vi "Open.vi"(8 "error in":errorcluster, 9 "parameters":variant, 10 "file path":path, 11 "cRIO repo in":refnum<class "cRIORepo.lvclass">) -> (0 "error out":errorcluster, 2 "invalid?":bool, 3 "cRIO repo out":refnum<class "cRIORepo.lvclass">)   [LabVIEW 2015, in "cRIORepo.lvclass"]
doc: "Here we are specifying to read the configuration from a gXML file. And version management"
uses:
  cRIORepo.lvclass
  FileCluster.ctl
  ChannelData.ctl
  cRIORepo.lvclass/cRIORepo.ctl
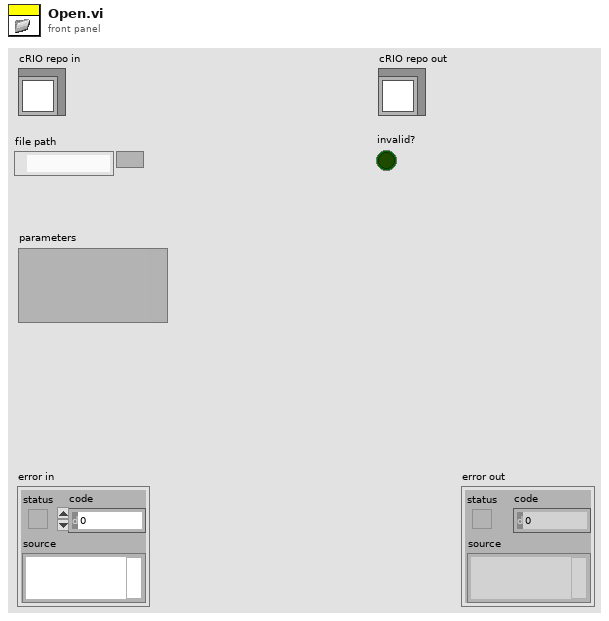
[diagram p1: front panel]
types:
  T1 = typedef "cRIORepo.lvclass/FileCluster.ctl" = cluster{"Version":string, "Data":variant}
  T2 = typedef "cRIORepo.lvclass/ChannelData.ctl" = cluster{"channel group":string, "channel name":string, "IO ":string, "sensor ID":string, "description":string, "system":string, "channel type":string}
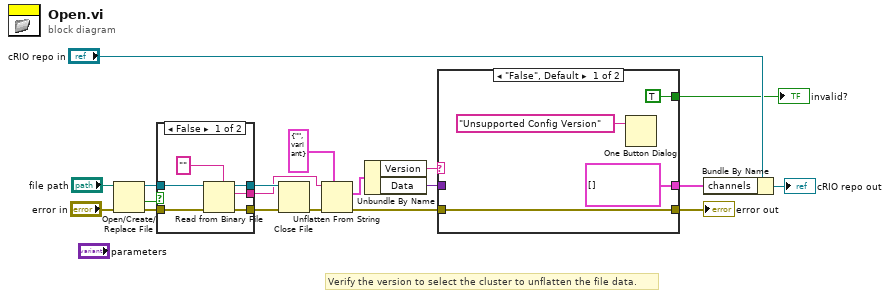
[diagram p0: block diagram]
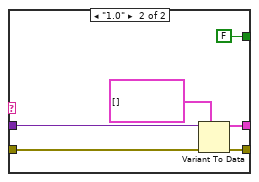
[diagram p2: hidden frame]
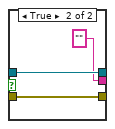
[diagram p3: hidden frame]
diagram:
  # "Verify the version to select the cluster to unflatten the file data."
  n1 = Open/Create/Replace File(file path (use dialog)="file path", error in="error in") -> (refnum out=w14:refnum<file>, cancelled=w15:bool, error out=w11:errorcluster)  [unwired: 4 in]
  n2 = case shown="False" w15 {
    tunnel: w14 -> [w25 w28]
    tunnel: [w24 w28] -> w13
    tunnel: [w23 w27] -> w12
    tunnel: w11 -> [w22 w27]
    tunnel: [w21 ""] -> w9
    frame False {
      n3 = Read from Binary File(5:"" ("data type"), 8:w22, 11:w25) -> (0:w23:errorcluster, 2:w21:string, 3:w24:refnum<file>)  [unwired: 3 in, 1 out]
    }
    frame True {
    }
  }
  n4 = Close File(refnum=w13, error in=w12) -> (error out=w5:errorcluster)  [unwired: 1 out]
  n5 = Unflatten From String(type=T1 {"Version"="", "Data"=variant}, binary string=w9, error in (no error)=w5) -> (value=w1:T1, error out=w6:errorcluster)  [unwired: 2 in, 1 out]
  n6 = Unbundle By Name(w1) -> ("Version"=w8:string, "Data"=w7:variant)
  n7 = case shown="\"False\", Default" w8 {
    tunnel: [T2[] [] ("channels") w37] -> w4
    tunnel: [w31 w36] -> w2
    tunnel: w6 -> [w31 w33]
    tunnel: w7 -> [_ w34]
    tunnel: [TRUE FALSE] -> w3
    frame "False", Default {
      n8 = One Button Dialog(message="Unsupported Config Version") -> ()  [unwired: 1 in, 1 out]
    }
    frame "1.0" {
      n9 = Variant To Data(error in=w33, type=T2[] [] ("channels"), Variant=w34) -> (data=w37:T2[], error out=w36:errorcluster)
    }
  }
  "error out" <- w2
  "invalid?" <- w3
  n10 = Bundle By Name(cluster="cRIO repo in", "channels"=w4) -> (→"cRIO repo out":refnum<class "cRIORepo.lvclass">)
